vi "KE2260B Configure Bleeder Circuit.vi"(8 "error in (no error)":errorcluster, 10 "Bleeder Circuit (T: Enable)":bool=TRUE, 11 "VISA resource name":refnum<visa-resource-name>) -> (0 "error out":errorcluster, 3 "VISA resource name out":refnum<visa-resource-name>)   [LabVIEW 2021, in "Keithley 2260B.lvlib"]
doc: "Turns the bleeder circuit on or off."
uses:
  Keithley 2260B.lvlib
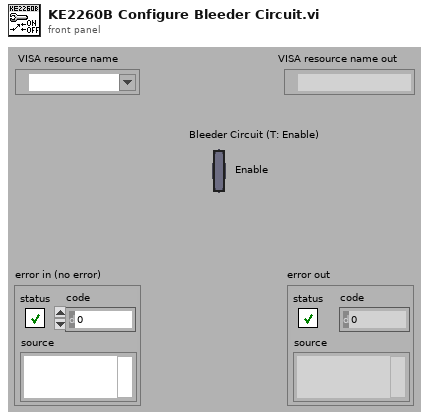
[diagram p1: front panel]
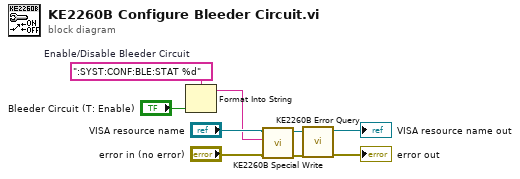
[diagram p0: block diagram]
diagram:
  w6 = ":SYST:CONF:BLE:STAT %d"  # Enable/Disable Bleeder Circuit
  n1 = Format Into String(format string=w6, "Bleeder Circuit (T: Enable)") -> (resulting string=w1:string)  [unwired: 2 in, 1 out]
  n2 = call "KE2260B Special Write.vi"("error in (no error)"="error in (no error)", "Write Buffer (\"\")"=w1, "VISA session"="VISA resource name") -> ("error out"=w5:errorcluster, "dup VISA session"=w4:refnum<visa-resource-name>)  [unwired: 6 in, 1 out]
  n3 = call "KE2260B Error Query.vi"("error in (no error)"=w5, "VISA resource name"=w4) -> ("error out"=→"error out":errorcluster, "VISA resource name out"=→"VISA resource name out":refnum<visa-resource-name>)  [unwired: 6 in, 2 out]
